vi "Get VI Clone Names.vi"(8 "error in (no error)":errorcluster, 11 "VI Ref":refnum<vi>) -> (0 "error out":errorcluster, 2 "Clone Names":string[](array[string]), 3 "VI Ref out":refnum<vi>)   [LabVIEW 2020, in "MacroAssert.lvlib"]
uses:
  MacroAssert.lvlib
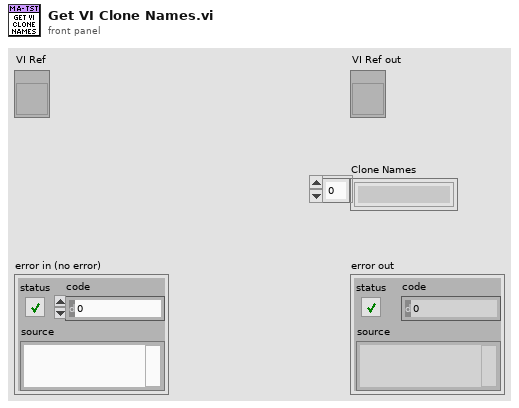
[diagram p1: front panel]
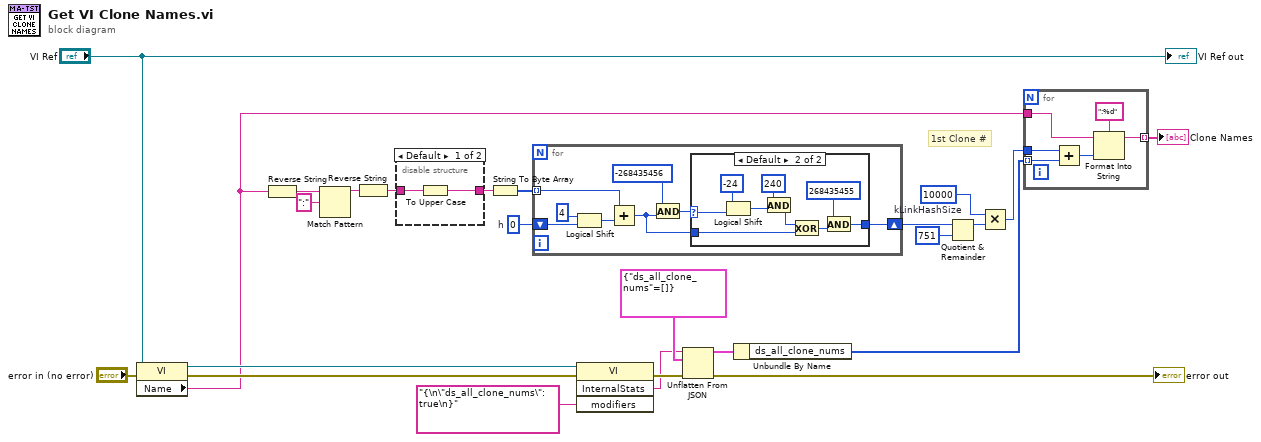
[diagram p0: block diagram]
diagram:
  w11 = 751  # kLinkHashSize
  w13 = 0  # h
  # "1st Clone #"
  n1 = property on="Property Node" class="VI"(reference="VI Ref", error in="error in (no error)") -> (reference out=w21:refnum<vi>, error out=w24:errorcluster, "Name"=w7:string)
  n2 = Reverse String(1:w7) -> (0:w17:string)
  n3 = Match Pattern(string=w17, regular expression=":") -> (before substring=w19:string)  [unwired: 1 in, 3 out]
  n4 = Reverse String(1:w19) -> (0:w16:string)
  n5 = disable-structure "Conditional Disable Structure" shown="Default" {
    disable-tunnel: w16 -> [w27 _]
    disable-tunnel: [w26 _] -> w15
    frame condition #0 (active) {
      n6 = To Upper Case(1:w27) -> (0:w26:string)
    }
    frame condition #1 {
    }
  }
  n7 = String To Byte Array(string=w15) -> (unsigned byte array=w14:u8[])
  n8 = for {
    tunnel: w14 -> [w32] mode=indexing
    shift-right: [w28] -> w12
    shift-left: w13 -> [w35]
    n9 = Logical Shift(y=4, x=w35) -> (x << y=w33:i32)
    n10 = Add(x=w32, y=w33) -> (x+y=w29:i32)
    n11 = And(x=-268435456, y=w29) -> (x .and. y?=w30:i32)
    n12 = case shown="Default" w30 {
      selector: w30 -> [_ w45]
      tunnel: w29 -> [w36 w40]
      tunnel: [w36 w37] -> w28
      frame 0 {
      }
      frame Default {
        n13 = Logical Shift(y=-24, x=w45) -> (x << y=w43:i32)
        n14 = And(x=240, y=w43) -> (x .and. y?=w41:i32)
        n15 = Exclusive Or(1:w40, 2:w41) -> (0:w38:i32)
        n16 = And(x=268435455, y=w38) -> (x .and. y?=w37:i32)
      }
    }
  }
  n17 = invoke class="VI" method="InternalStats"(reference=w21, error in=w24, "modifiers"="{\n\"ds_all_clone_nums\": true\n}") -> (error out=w25:errorcluster, "InternalStats"=w2:string)  [unwired: 1 in, 2 out]
  n18 = Unflatten From JSON(JSON string=w2, type and defaults=cluster{"ds_all_clone_nums":i32[]} {"ds_all_clone_nums"=[]}, error in (no error)=w25) -> (value=w3:cluster{"ds_all_clone_nums":i32[]}, error out=→"error out":errorcluster)  [unwired: 4 in]
  n19 = Unbundle By Name(w3) -> ("ds_all_clone_nums"=w6:i32[])
  n20 = Quotient & Remainder(x=w12, y=w11) -> (x-y*floor(x/y)=w10:i32)  [unwired: 1 out]
  n21 = Multiply(x=10000, y=w10) -> (x*y=w8:i32)
  n22 = for {
    tunnel: [w51] -> w1 mode=indexing
    tunnel: w8 -> [w50]
    tunnel: w7 -> [w49]
    tunnel: w6 -> [w48] mode=indexing
    n23 = Add(x=w50, y=w48) -> (x+y=w47:i32)
    n24 = Format Into String(format string=":%d", initial string=w49, w47) -> (resulting string=w51:string)  [unwired: 1 in, 1 out]
  }
  "Clone Names" <- w1
  "VI Ref out" <- "VI Ref"
